vi "Full Force Test DAA.vi"(8 "error in (no error)":errorcluster, 10 "Model in":refnum<class "Model.lvclass">, 11 "Test Actuator State in":refnum<class "Test Actuator State.lvclass">) -> (0 "error out":errorcluster, 1 "Pass":bool, 2 "Model out":refnum<class "Model.lvclass">, 3 "Test Actuator State out":refnum<class "Test Actuator State.lvclass">)   [LabVIEW 2016]
uses:
  Model/Model/Model.lvclass
  Typedefs/ActuatorSetPoints.ctl
  <vilib>/platform/TimedLoop/XDataNode/XDataNode.xnode
  <vilib>/Platform/TimedLoop/XDataNode/nitl_modes.ctl
  <vilib>/Platform/TimedLoop/XDataNode/XDNodeRunTimeDep.lvlib
  <vilib>/Platform/TimedLoop/XDataNode/wakeup.ctl
  <vilib>/Platform/TimedLoop/XDataNode/timing_clust.ctl
  Test Actuator State.lvclass
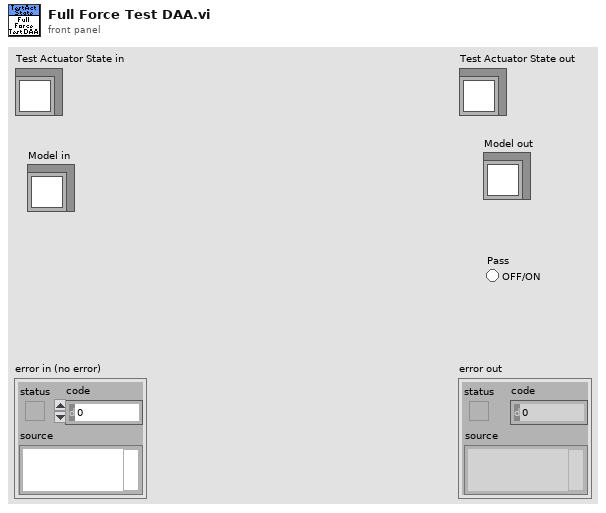
[diagram p1: front panel]
types:
  T1 = typedef "FullForceScanSettings.ctl" = cluster{"Force Tolerance (N)":dbl, "DAA Force Set Points":T2[], "Process Time (s)":dbl, "Sample Time (s)":dbl, "Max Moment (NM)":dbl, "SAA Force Set Points":T2[]}
  T2 = typedef "ForcePair.ctl" = cluster{"Axial Force":dbl, "Lateral Force":dbl}
  T3 = typedef "ActuatorSetPoints.ctl" = cluster{"Axial Force":dbl, "Lateral Force":dbl, "FC1 Force":dbl, "FC2 Force":dbl}
  T4 = typedef "XDNodeRunTimeDep.lvlib/timing_clust.ctl" = cluster{"Expected End [f-1]":u64, "Actual End [f-1]":u64, "Finished Late? [f-1]":bool, "Expected End [i-1]":u64, "Actual End [i-1]":u64, "Finished Late? [i-1]":bool, "Expected Start [i]":u64, "Actual Start [i]":u64, "Expected Start [f]":u64, "Actual Start [f]":u64, "Source Name":string, "Structure Name":string, "Period":i64, "Deadline":i64, "Offset":i64, "Start":i64, "Priority":i32, "Timeout":i32, "Mode":T5, "Wakeup Reason":T6, "Error":errorcluster, "Source Type":string, "Secondary Source Type":string, "Global End Time":u64, "Global Start Time":u64, "Frame Duration":u64, "Iteration Duration":u64, "Assigned CPU":i32, "I/O Scan Engine Mode":u32}
  T5 = typedef "XDNodeRunTimeDep.lvlib/nitl_modes.ctl" = enum32{"No Change", "Process missed periods, maintain original phase", "Discard missed periods, maintain original phase", "Process missed periods, ignore original phase", "Discard missed periods, ignore original phase"}
  T6 = typedef "XDNodeRunTimeDep.lvlib/wakeup.ctl" = enum32{"Normal", "Aborted", "Asynchronous wakeup", "Timing source error", "Timed loop error", "Timeout"}
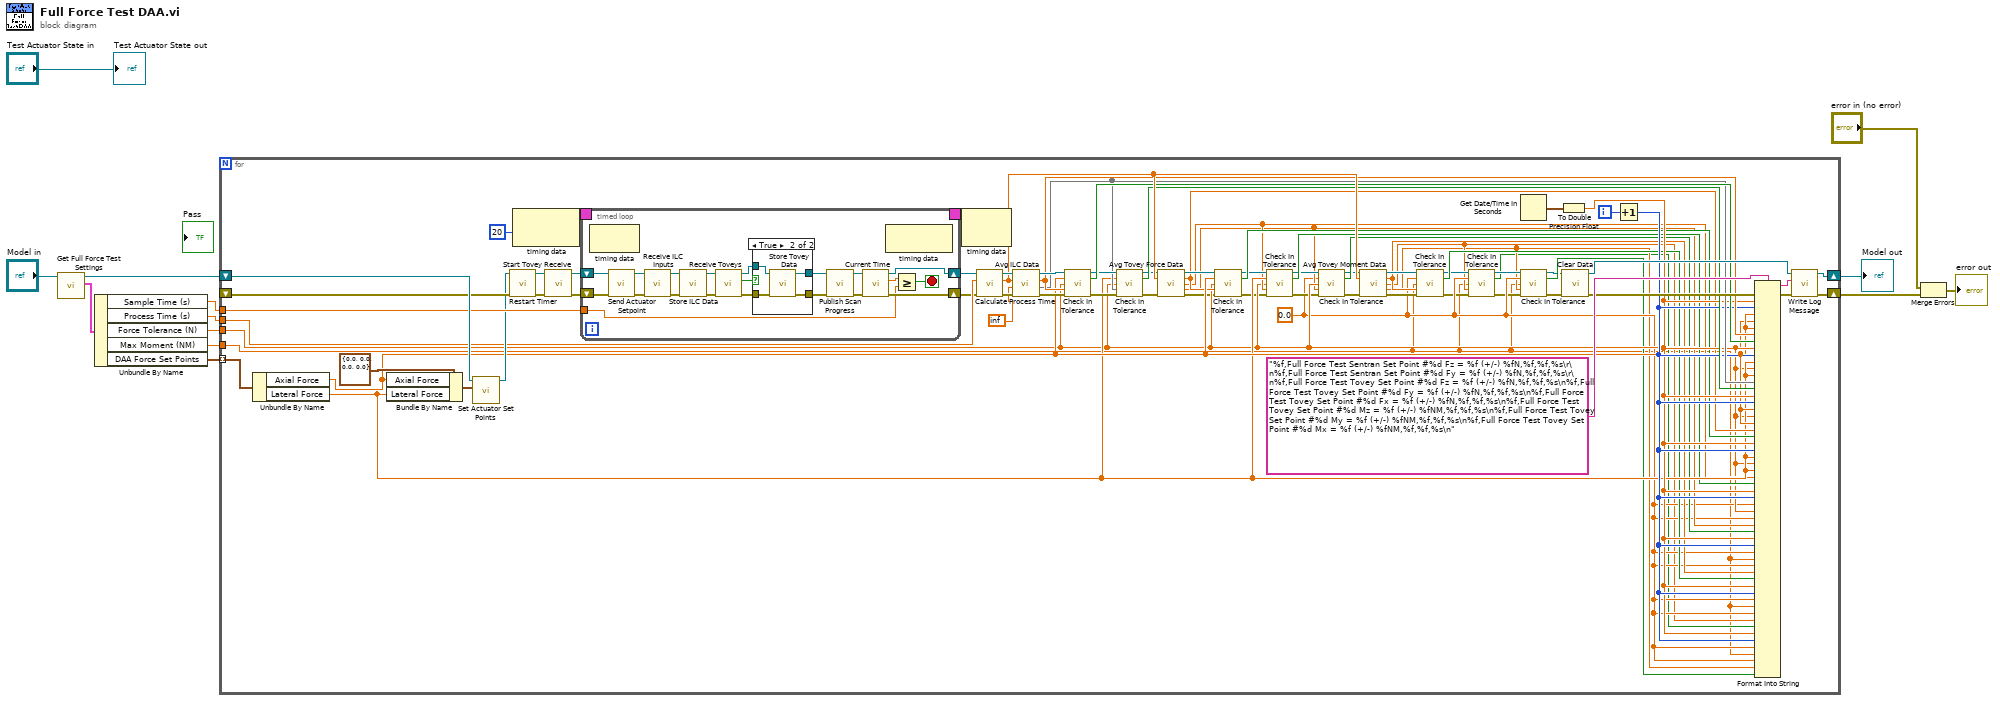
[diagram p0: block diagram]
diagram:
  n1 = call "Get Full Force Test Settings.vi"("Model in"="Model in") -> ("Full Force Test Settings"=w2:T1, "Model out"=w12:refnum<class "Model.lvclass">)  [unwired: 9 in]
  n2 = Unbundle By Name(w2) -> ("Sample Time (s)"=w11:dbl, "Process Time (s)"=w10:dbl, "Force Tolerance (N)"=w9:dbl, "Max Moment (NM)"=w4:dbl, "DAA Force Set Points"=w1:T2[])
  n3 = for {
    tunnel: w1 -> [w73] mode=indexing
    shift-right: [w83] -> w6
    shift-left: w12 -> [w87]
    tunnel: w11 -> [w86]
    tunnel: w10 -> [w68]
    tunnel: w9 -> [w41]
    shift-right: [w69] -> w5
    shift-left: _ -> [w85]
    tunnel: w4 -> [w18]
    i -> [w80]
    w27 = 0.0
    n4 = Unbundle By Name(w73) -> ("Axial Force"=w49:dbl, "Lateral Force"=w45:dbl)
    n5 = Bundle By Name(cluster=T3 {"Axial Force"=0.0, "Lateral Force"=0.0, "FC1 Force"=0.0, "FC2 Force"=0.0} ("Actuator Set Points"), "Axial Force"=w49, "Lateral Force"=w45) -> (w74:T3)
    n6 = call "Set Actuator Set Points.vi"("Actuator Set Points"=w74, "Model in"=w87) -> ("Model out"=w75:refnum<class "Model.lvclass">)  [unwired: 9 in]
    n7 = call "Restart Timer.vi"("error in (no error)"=w85, "Model in"=w75) -> ("error out"=w78:errorcluster, "Model out"=w79:refnum<class "Model.lvclass">)  [unwired: 8 in]
    n8 = node-c288(i64 20 ("Period")) -> (w16:T4)
    n9 = call "Start Tovey Receive.vi"("error in (no error)"=w78, "Model in"=w79) -> ("error out"=w76:errorcluster, "Model out"=w77:refnum<class "Model.lvclass">)  [unwired: 8 in]
    n10 = timed-loop {
      shift-right: [w102] -> w67
      shift-left: w77 -> [w108]
      shift-right: [w101] -> w65
      shift-left: w76 -> [w105]
      tunnel: w86 -> [w99]
      timing: w16 -> [_]
      timing-out: [_] -> w15
      stop <- w98 stop-if-true
      n11 = node-c288() -> ()  [unwired: 1 in, 1 out]
      n12 = call "Send Actuator Setpoint.vi"("error in (no error)"=w105, "Model in"=w108) -> ("error out"=w104:errorcluster, "Model out"=w107:refnum<class "Model.lvclass">)  [unwired: 8 in]
      n13 = call "Receive ILC Inputs.vi"("error in (no error)"=w104, "Model in"=w107) -> ("error out"=w103:errorcluster, "Model out"=w106:refnum<class "Model.lvclass">)  [unwired: 8 in]
      n14 = call "Store ILC Data.vi"("error in (no error)"=w103, "Model in"=w106) -> ("error out"=w96:errorcluster, "Model out"=w97:refnum<class "Model.lvclass">)  [unwired: 8 in]
      n15 = call "Receive Toveys.vi"("error in (no error)"=w96, "Model in"=w97) -> ("error out"=w94:errorcluster, "Data Received"=w93:bool, "Model out"=w95:refnum<class "Model.lvclass">)  [unwired: 7 in]
      n16 = case shown="True" w93 {
        tunnel: w95 -> [w112 w116]
        tunnel: w94 -> [w111 w115]
        tunnel: [w111 w114] -> w89
        tunnel: [w112 w113] -> w92
        frame False {
        }
        frame True {
          n17 = call "Store Tovey Data.vi"("error in (no error)"=w115, "Model in"=w116) -> ("error out"=w114:errorcluster, "Model out"=w113:refnum<class "Model.lvclass">)  [unwired: 8 in]
        }
      }
      n18 = call "Publish Scan Progress.vi"("error in (no error)"=w89, "Model in"=w92) -> ("error out"=w90:errorcluster, "Model out"=w91:refnum<class "Model.lvclass">)  [unwired: 8 in]
      n19 = call "Current Time.vi"("error in (no error)"=w90, "Model in"=w91) -> ("error out"=w101:errorcluster, "Time"=w100:dbl, "Model out"=w102:refnum<class "Model.lvclass">)  [unwired: 7 in]
      n20 = node-c288() -> ()  [unwired: 1 in, 1 out]
      n21 = Greater Or Equal?(x=w100, y=w99) -> (x >= y?=w98:bool)
    }
    n22 = node-c288(w15) -> ()  [unwired: 1 out]
    n23 = call "Calculate Process Time.vi"("error in (no error)"=w65, "Seconds"=w68, "Model in"=w67) -> ("error out"=w64:errorcluster, "Time"=w63:dbl, "Model out"=w66:refnum<class "Model.lvclass">)  [unwired: 6 in]
    n24 = call "Avg ILC Data.vi"("error in (no error)"=w64, "Before This Time"=inf, "After This Time"=w63, "Model in"=w66) -> ("error out"=w56:errorcluster, 1:w58, "Force"=w61:dbl, "Model out"=w62:refnum<class "Model.lvclass">)  [unwired: 4 in]
    n25 = call "Check In Tolerance.vi"("Model in"=w62, "Expected"=w49, "Tolerance"=w41, "Actual"=w61, "error in (no error)"=w56) -> ("Model out"=w59:refnum<class "Model.lvclass">, "Pass"=w60:bool, "error out"=w55:errorcluster)  [unwired: 8 in]
    n26 = call "Check In Tolerance.vi"("Model in"=w59, "Expected"=w45, "Tolerance"=w41, "Actual"=w58, "error in (no error)"=w55) -> ("Model out"=w53:refnum<class "Model.lvclass">, "Pass"=w57:bool, "error out"=w54:errorcluster)  [unwired: 8 in]
    n27 = call "Avg Tovey Force Data.vi"("Model in"=w53, "After This Time"=w63, "error in (no error)"=w54) -> ("Model out"=w50:refnum<class "Model.lvclass">, "Fz"=w47:dbl, "Fy"=w43:dbl, "Fx"=w31:dbl, "error out"=w38:errorcluster)  [unwired: 8 in]
    n28 = call "Check In Tolerance.vi"("Model in"=w50, "Expected"=w49, "Tolerance"=w41, "Actual"=w47, "error in (no error)"=w38) -> ("Model out"=w46:refnum<class "Model.lvclass">, "Pass"=w48:bool, "error out"=w37:errorcluster)  [unwired: 8 in]
    n29 = call "Check In Tolerance.vi"("Model in"=w46, "Expected"=w45, "Tolerance"=w41, "Actual"=w43, "error in (no error)"=w37) -> ("Model out"=w42:refnum<class "Model.lvclass">, "Pass"=w44:bool, "error out"=w36:errorcluster)  [unwired: 8 in]
    n30 = call "Check In Tolerance.vi"("Model in"=w42, "Expected"=w27, "Tolerance"=w41, "Actual"=w31, "error in (no error)"=w36) -> ("Model out"=w34:refnum<class "Model.lvclass">, "Pass"=w40:bool, "error out"=w35:errorcluster)  [unwired: 8 in]
    n31 = call "Avg Tovey Moment Data.vi"("Model in"=w34, "After This Time"=w63, "error in (no error)"=w35) -> ("Model out"=w33:refnum<class "Model.lvclass">, "Mz"=w30:dbl, "My"=w26:dbl, "Mx"=w25:dbl, "error out"=w32:errorcluster)  [unwired: 8 in]
    n32 = call "Check In Tolerance.vi"("Model in"=w33, "Expected"=w27, "Tolerance"=w18, "Actual"=w30, "error in (no error)"=w32) -> ("Model out"=w29:refnum<class "Model.lvclass">, "Pass"=w39:bool, "error out"=w21:errorcluster)  [unwired: 8 in]
    n33 = call "Check In Tolerance.vi"("Model in"=w29, "Expected"=w27, "Tolerance"=w18, "Actual"=w26, "error in (no error)"=w21) -> ("Model out"=w28:refnum<class "Model.lvclass">, "Pass"=w24:bool, "error out"=w20:errorcluster)  [unwired: 8 in]
    n34 = Get Date/Time In Seconds() -> (seconds since 1Jan1904=w81:timestamp)
    n35 = call "Check In Tolerance.vi"("Model in"=w28, "Expected"=w27, "Tolerance"=w18, "Actual"=w25, "error in (no error)"=w20) -> ("Model out"=w22:refnum<class "Model.lvclass">, "Pass"=w23:bool, "error out"=w19:errorcluster)  [unwired: 8 in]
    n36 = To Double Precision Float(number=w81) -> (double precision float=w51:dbl)
    n37 = call "Clear Data.vi"("error in (no error)"=w19, "Model in"=w22) -> ("error out"=w71:errorcluster, "Model out"=w84:refnum<class "Model.lvclass">)  [unwired: 8 in]
    n38 = Increment(x=w80) -> (x+1=w52:i32)
    n39 = Format Into String(format string="%f,Full Force Test Sentran Set Point #%d Fz = %f (+/-) %fN,%f,%f,%s\r\n%f,Full Force Test Sentran Set Point #%d Fy = %f (+/-) %fN,%f,%f,%s\r\n%f,Full Force Test Tovey Set Point #%d Fz = %f (+/-) %fN,%f,%f,%s\n%f,Full Force Test Tovey Set Point #%d Fy = %f (+/-) %fN,%f,%f,%s\n%f,Full Force Test Tovey Set Point #%d Fx = %f (+/-) %fN,%f,%f,%s\n%f,Full Force Test Tovey Set Point #%d Mz = %f (+/-) %fNM,%f,%f,%s\n%f,Full Force Test Tovey Set Point #%d My = %f (+/-) %fNM,%f,%f,%s\n%f,Full Force Test Tovey Set Point #%d Mx = %f (+/-) %fNM,%f,%f,%s\n", error in=w71, w51, w52, w49, w41, w49, w61, w60, w51, w52, w45, w41, w45, w58, w57, w51, w52, w49, w41, w49, w47, w48, w51, w52, w45, w41, w45, w43, w44, w51, w52, w27, w41, w27, w31, w40, w51, w52, w27, w18, w27, w30, w39, w51, w52, w27, w18, w27, w26, w24, w51, w52, w27, w18, w27, w25, w23) -> (resulting string=w72:string, error out=w70:errorcluster)  [unwired: 1 in]
    n40 = call "Write Log Message.vi"("error in (no error)"=w70, "Message"=w72, "Model in"=w84) -> ("error out"=w69:errorcluster, "Model out"=w83:refnum<class "Model.lvclass">)  [unwired: 7 in]
  }
  "Model out" <- w6
  n41 = Merge Errors("error in (no error)", w5) -> (→"error out":errorcluster)
  "Test Actuator State out" <- "Test Actuator State in"
